vi "PROVA VIBRAZIONI.vi"() -> ()   [LabVIEW 2019]
uses:
  <vilib>/DAQmx/read.llb/DAQmx Read (Analog Wfm 1Chan NSamp).vi
  <vilib>/DAQmx/create/channels.llb/DAQmx Create Channel (AI-Acceleration-Accelerometer).vi
  <vilib>/DAQmx/configure/timing.llb/DAQmx Timing (Sample Clock).vi
  <vilib>/DAQmx/miscellaneous.llb/DAQmx Fill In Error Info.vi
  <vilib>/measure/matone.llb/Harmonic Distortion Analyzer 1 Chan.vi
  <vilib>/measure/maspectr.llb/FFT Spectrum (Mag-Phase) for 1 Chan.vi
  <vilib>/measure/NI_MAPro.lvlib
panel:
  in  "measurement info":T1={"uncertainty"=0.0, "Warning"=FALSE, "comments"="reserved for future use"} {"uncertainty" format="%0.2p"}
  in  "Cluster":T2
  out "RPM":dbl
  out "detected fundamental frequency":dbl format="%.2p"
  in  "stop":bool
  out "Waveform Graph":waveform(dbl)(graph)
  in  "number of samples per channel":i32=-1
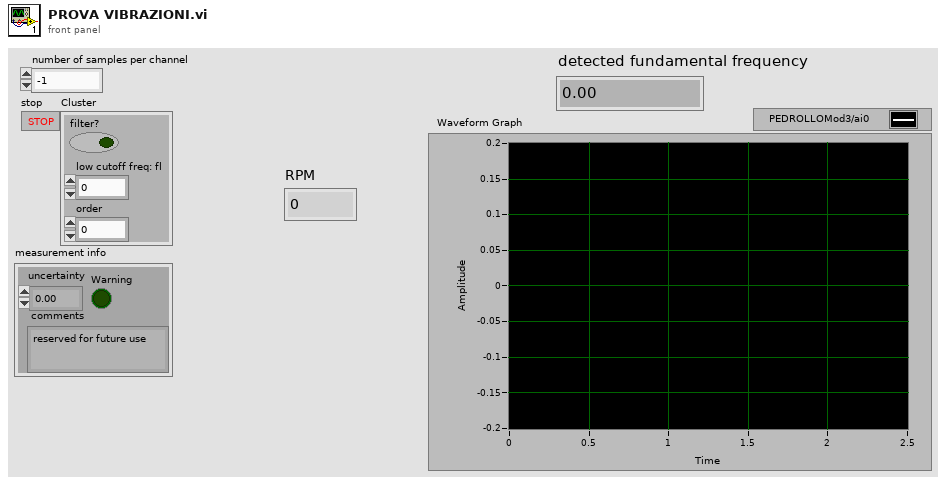
[diagram p1: front panel]
types:
  T1 = cluster{"uncertainty":dbl, "Warning":bool, "comments":string}
  T2 = cluster{"filter?":bool, "low cutoff freq: fl":dbl, "order":i32}
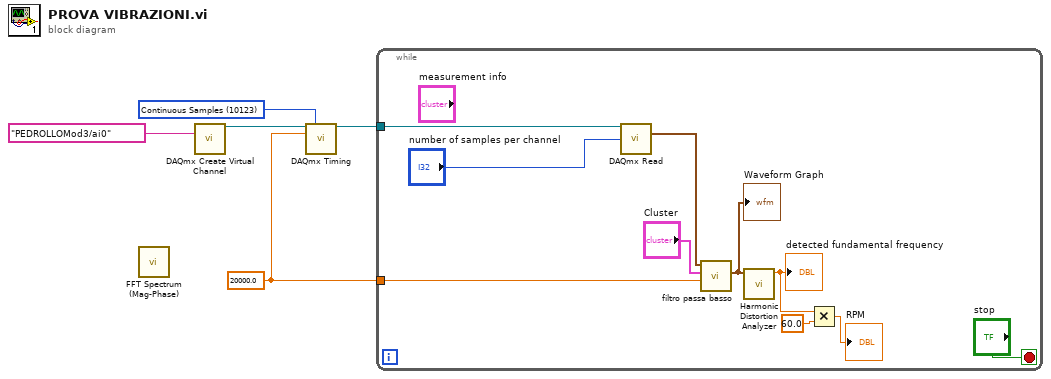
[diagram p0: block diagram]
diagram:
  w1 = 20000.0 ("rate")
  w3 = 10123 items=["Finite Samples"=10178, "Continuous Samples"=10123, "Hardware Timed Single Point"=12522] ("sample mode")
  n1 = call-poly <vilib>:"FFT Spectrum (Mag-Phase).vi"() -> ()  [unwired: 7 in, 5 out]
  n2 = call-poly <vilib>:"DAQmx Create Virtual Channel.vi"("physical channels"=tag "PEDROLLOMod3/ai0") -> ("task out"=w4:refnum<k21>)  [unwired: 13 in, 1 out]
  n3 = call-poly <vilib>:"DAQmx Timing.vi"("task/channels in"=w4, "sample mode"=w3, "rate"=w1) -> ("task out"=w2:refnum<k21>)  [unwired: 11 in, 1 out]
  n4 = while {
    tunnel: w2 -> [w15]
    tunnel: w1 -> [w7]
    stop <- "stop" stop-if-true
    n5 = call-poly <vilib>:"DAQmx Read.vi"("task/channels in"=w15, "number of samples per channel"="number of samples per channel") -> ("data"=w9:waveform(dbl))  [unwired: 11 in, 2 out]
    n6 = call "filtro passa basso.vi"("sampling freq: fs"=w7, "Cluster"="Cluster", "Waveform"=w9) -> ("Waveform 2"=w6:waveform(dbl))  [unwired: 8 in]
    "Waveform Graph" <- w6
    n7 = call-poly <vilib>:"Harmonic Distortion Analyzer.vi"("signal in"=w6) -> ("detected fundamental frequency"=w12:dbl)  [unwired: 5 in, 5 out]
    "detected fundamental frequency" <- w12
    n8 = Multiply(x=w12, y=60.0) -> (x*y=→"RPM":dbl)
  }
